vi "Main UI.vi"() -> ()   [LabVIEW 2017]
uses:
  UI typedefs/Controller Commands.ctl
  UI typedefs/Progress States.ctl
  Application Utilities/Console Log/Console Log.lvclass
  Procedure Classes/Potting Procedure/Potting Procedure.lvclass
  Shared Components/Gantry Class/Gantry Class.lvclass
  C:/Program Files/National Instruments/LabVIEW 2017/user.lib/aerotech/2010/Bin/Aerotech.A3200.dll
  Program Files/National Instruments/LabVIEW 2017/user.lib/aerotech/2010/Bin/Aerotech.A3200.dll
  Shared Components/WorkTable Class/Type Definitions/Worktable_Mode.ctl
  Shared Components/Gantry Class/Type Definitions/Virtual Modes.ctl
  UI typedefs/Progress Bar.ctl
panel:
  in  "ESTOP References":T1
  out "Progress":T2 scale=0.0..9.0
  in  "Execute Step":bool
  in  "Resume Button":bool
  in  "Suspend Button":bool
  in  "Add Comment":bool
  in  "Comment":string
  in  "Previous Button":bool
  in  "Manual Control":bool
  in  "Emergency Stop":bool
  out "Console":string
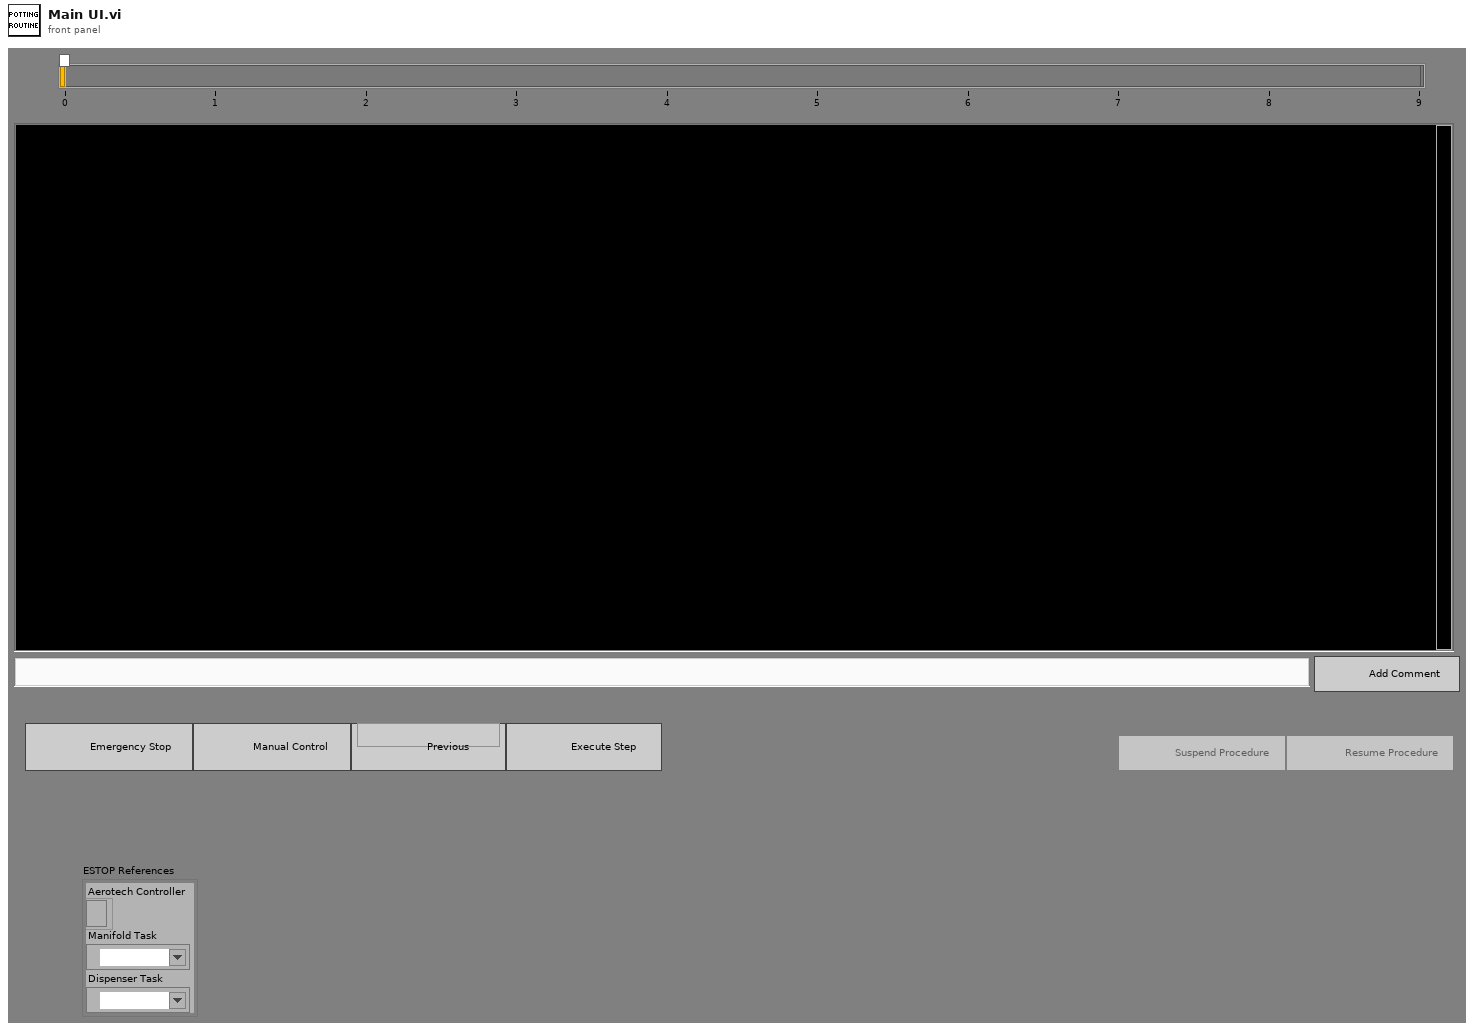
[diagram p1: front panel]
types:
  T1 = cluster{"Aerotech Controller":refnum<k24>, "Manifold Task":refnum<k21>, "Dispenser Task":refnum<k21>}
  T2 = typedef "Progress Bar.ctl" = u16
  T3 = typedef "Progress States.ctl" = enum16{"Configure Tester", "Inspect Fiducials", "Review Fiducials", "Inspect Modules", "Review Modules", "Fill Sylgard", "Align Needle", "Purge", "Pot", "Finish"}
  T4 = typedef "Controller Commands.ctl" = enum16{"Initialize", "Execute Step", "Previous Step", "Add Comment", "Manual Control", "Resume", "Pause", "Emergency Stop"}
  T5 = typedef "Virtual Modes.ctl" = enum16{"Nonvirtual", "Virtual"}
  T6 = typedef "Worktable_Mode.ctl" = enum16{"Encapsulation", "Gluing"}
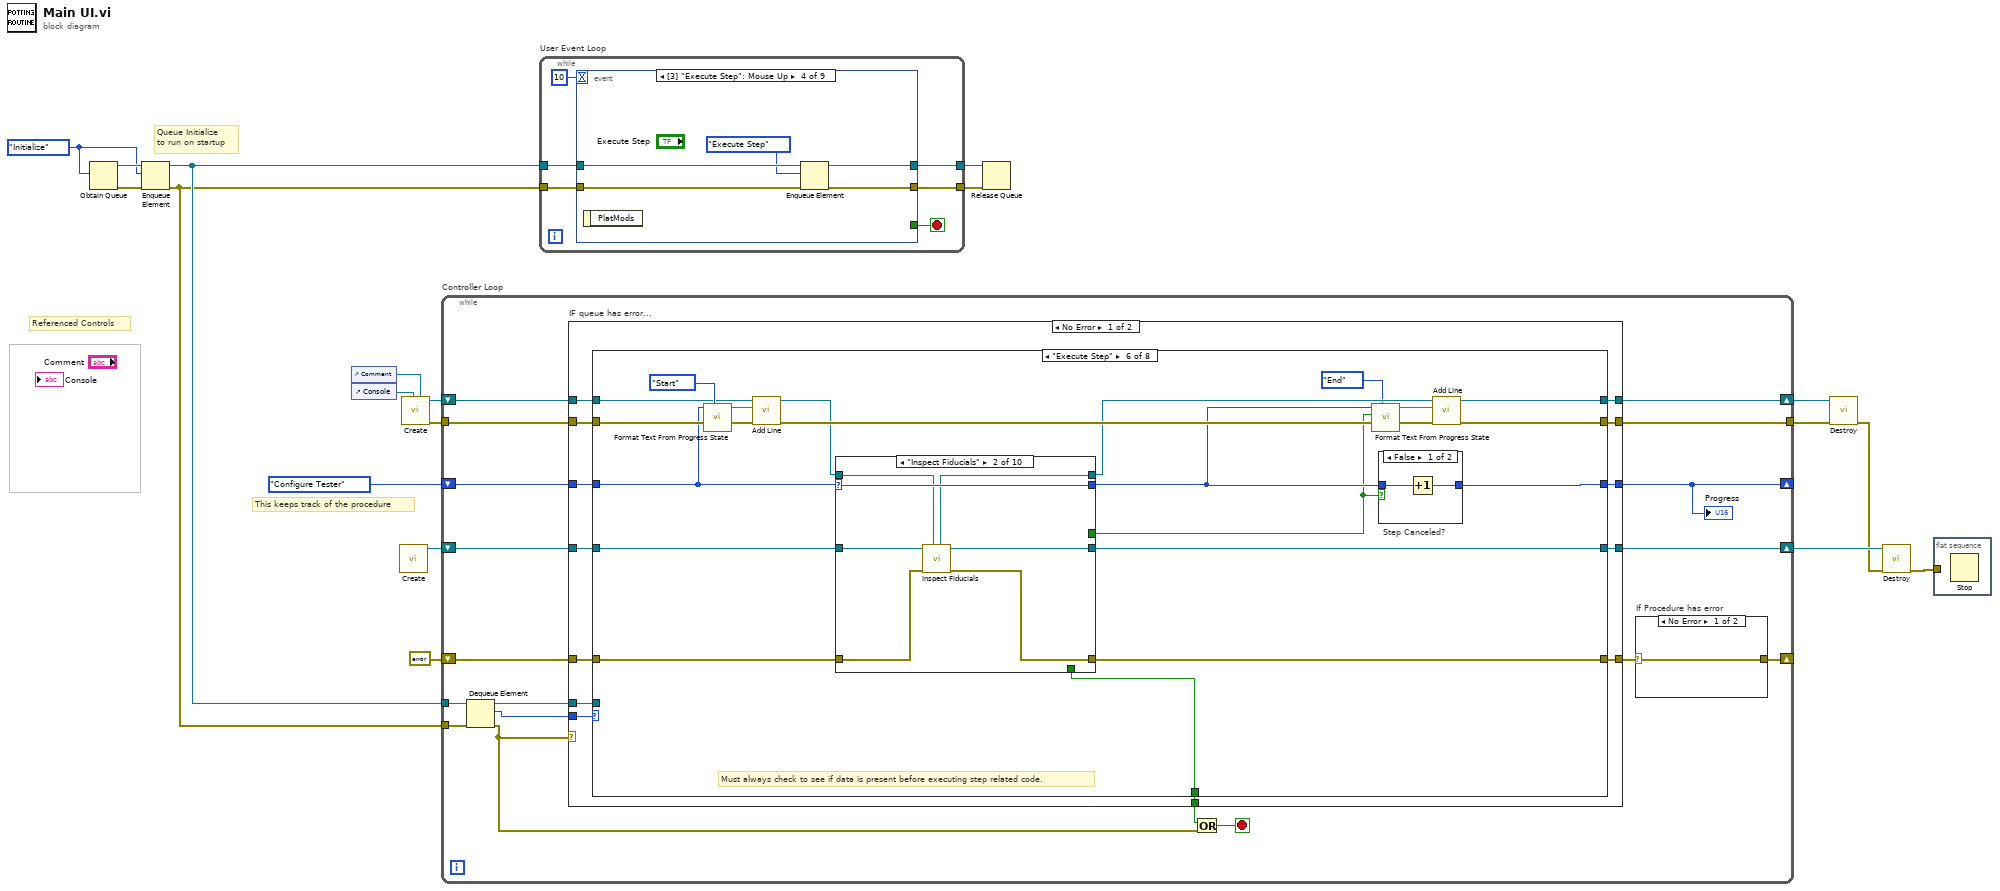
[diagram p0: block diagram]
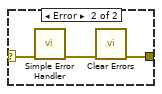
[diagram p2: hidden frame]
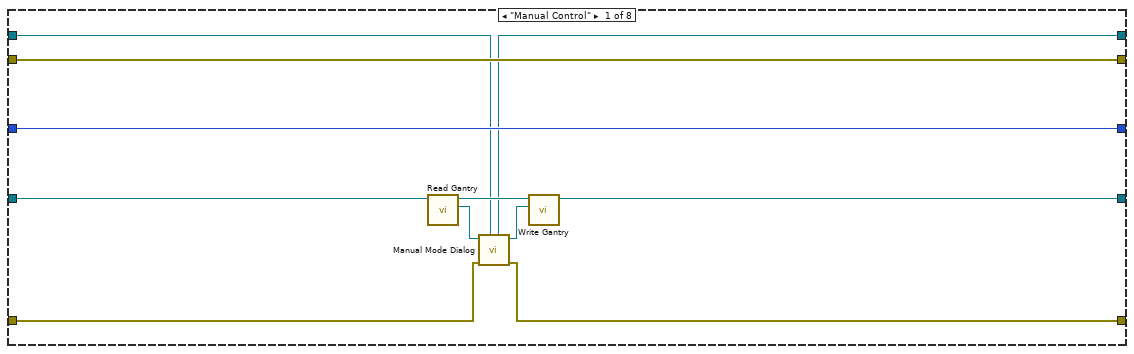
[diagram p3: hidden frame]
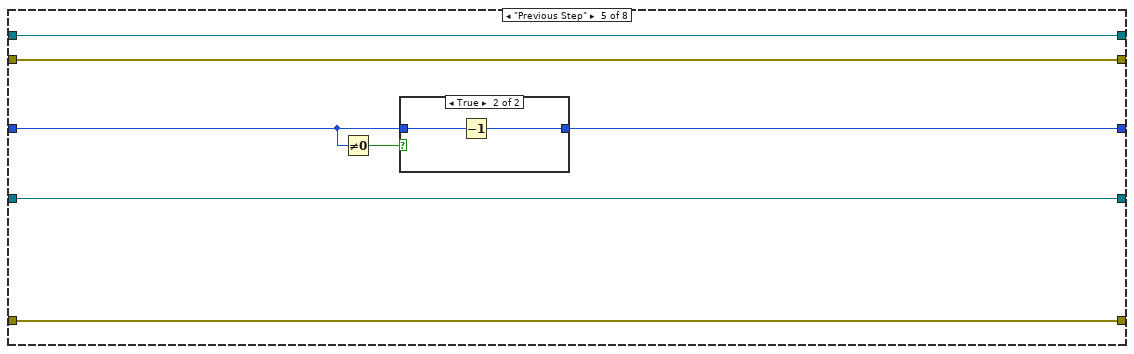
[diagram p7: hidden frame]
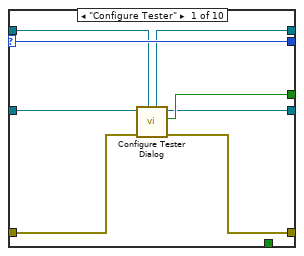
[diagram p10: hidden frame]
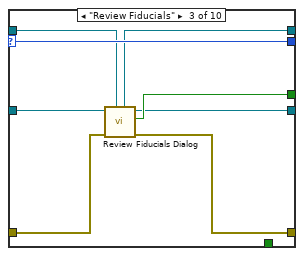
[diagram p11: hidden frame]
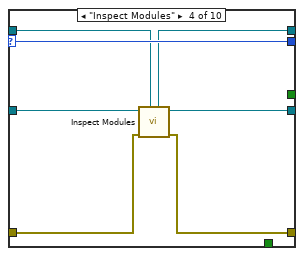
[diagram p12: hidden frame]
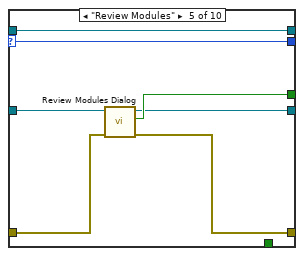
[diagram p13: hidden frame]
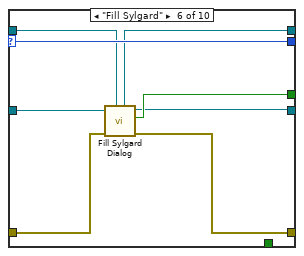
[diagram p14: hidden frame]
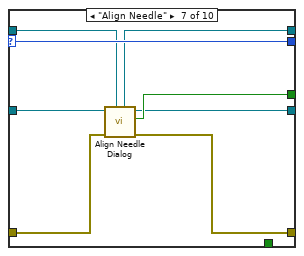
[diagram p15: hidden frame]
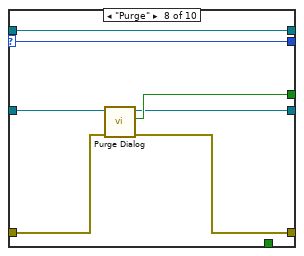
[diagram p16: hidden frame]
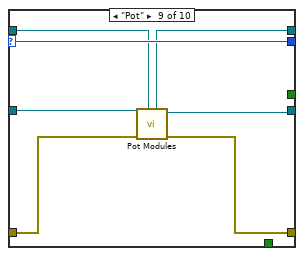
[diagram p17: hidden frame]
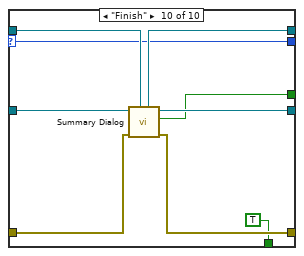
[diagram p18: hidden frame]
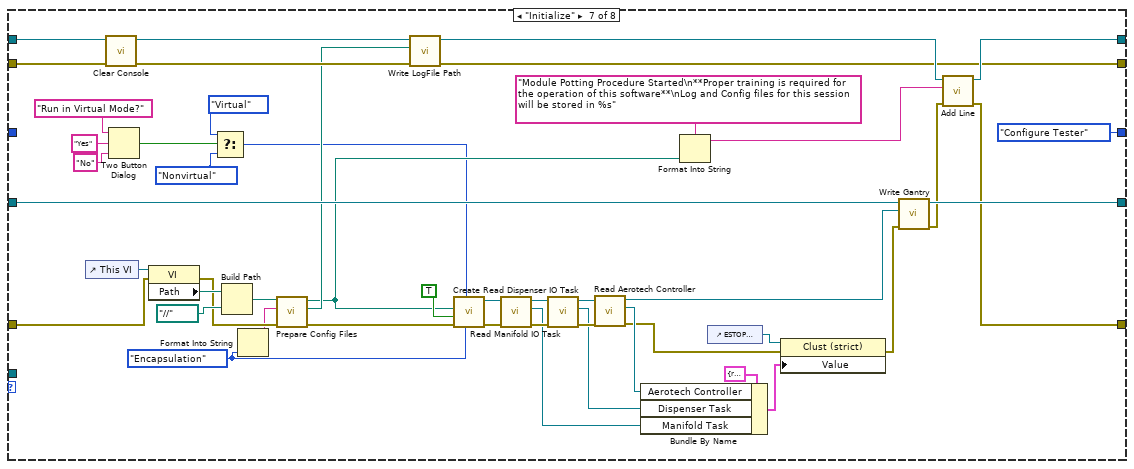
[diagram p19: hidden frame]
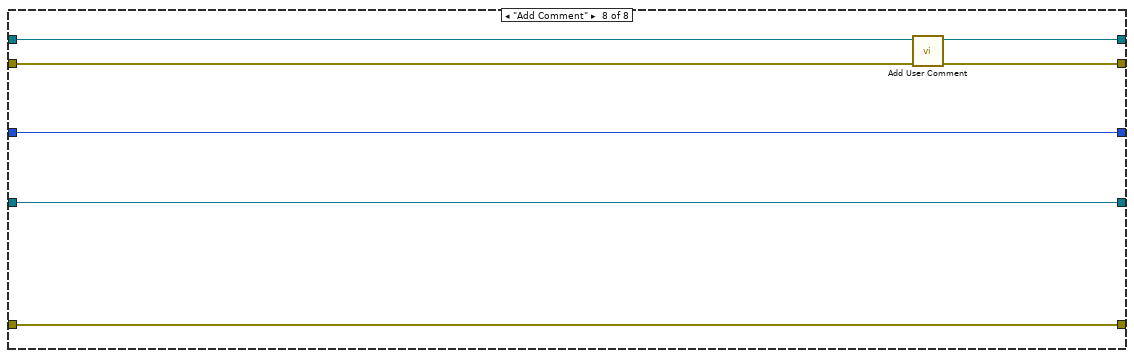
[diagram p20: hidden frame]
diagram:
  w12 = Controller_Commands."Initialize" ("Commands")
  # "Referenced Controls"
  # "This keeps track of the procedure"
  # "Queue Initialize \nto run on startup"
  n1 = Obtain Queue(element data type=w12) -> (queue out=w15:refnum<queue>, error out=w13:errorcluster)  [unwired: 4 in, 1 out]
  n2 = Enqueue Element(queue=w15, element=w12, error in (no error)=w13) -> (queue out=w14:refnum<queue>, error out=w1:errorcluster)  [unwired: 1 in, 1 out]
  n3 = control-ref of="Comment"() -> (w10:refnum<vi>)
  n4 = control-ref of="Console"() -> (w11:refnum<vi>)
  n5 = call "Create.vi"() -> ("Potting Procedure out"=w5:refnum<class "Potting Procedure.lvclass">)  [unwired: 10 in, 1 out]
  n6 = call "Create.vi"("Comment"=w10, "Console"=w11) -> ("error out"=w8:errorcluster, "Console Log out"=w9:refnum<class "Console Log.lvclass">)  [unwired: 8 in]
  n7 = while "Controller Loop" {
    tunnel: w1 -> [w37]
    shift-right: [w20] -> _
    shift-left: Progress_States."Configure Tester" -> [w35]
    tunnel: w14 -> [w34]
    shift-right: [w30] -> _
    shift-left: errorcluster {"status"=FALSE, "code"=0, "source"=""} ("error constant") -> [w32]
    tunnel: w8 -> [w27]
    tunnel: [w26] -> w6
    shift-right: [w28] -> w7
    shift-left: w9 -> [w29]
    shift-right: [w24] -> w4
    shift-left: w5 -> [w25]
    stop <- w22 stop-if-true
    n8 = Dequeue Element(queue=w34, error in (no error)=w37) -> (queue out=w36:refnum<queue>, element=w33:T4, error out=w23:errorcluster)  [unwired: 1 in, 1 out]
    n9 = case "IF queue has error..." shown="No Error" w23 {
      tunnel: w36 -> [w54 _]
      tunnel: w35 -> [w53 w248]
      tunnel: [w52 w248] -> w20
      tunnel: w33 -> [w51 _]
      tunnel: w32 -> [w50 w247]
      tunnel: [w49 w247] -> w31
      tunnel: w29 -> [w48 w246]
      tunnel: [w47 w246] -> w28
      tunnel: w27 -> [w46 w245]
      tunnel: [w45 w245] -> w26
      tunnel: [w43 w244] -> w24
      tunnel: w25 -> [w44 w244]
      tunnel: [w42 _] -> w21
      frame No Error {
        n10 = case shown="\"Execute Step\"" w51 {
          tunnel: w54 -> [_ _ _ _ _ _ _ _]
          tunnel: w53 -> [w65 w70 w75 w80 w82 w92 _ w243]
          tunnel: [w65 w70 w75 w80 w86 w109 Progress_States."Configure Tester" w243] -> w52
          tunnel: w50 -> [w63 w69 w74 w79 w87 w99 w200 w238]
          tunnel: [w62 w69 w74 w79 w87 w98 w210 w238] -> w49
          tunnel: w48 -> [w56 w67 w73 w78 w85 w94 w235 w240]
          tunnel: [w55 w67 w73 w78 w85 w108 w212 w242] -> w47
          tunnel: w46 -> [w64 w68 w72 w77 w84 w107 w234 w239]
          tunnel: [w64 w68 w72 w77 w84 w106 w206 w241] -> w45
          tunnel: w44 -> [w59 w66 w71 w76 w83 w103 w233 w237]
          tunnel: [w57 w66 w71 w76 w83 w102 w232 w237] -> w43
          tunnel: [_ _ _ _ _ w100 _ _] -> w42
          frame "Manual Control" {
            n11 = call-dynamic "Read Gantry.vi"("Potting Procedure in"=w59) -> ("Gantry"=w61:refnum<class "Gantry Class.lvclass">, "Potting Procedure out"=w58:refnum<class "Potting Procedure.lvclass">)  [unwired: 8 in, 1 out]
            n12 = call "Manual Mode Dialog.vi"("Console Log in"=w56, "error in"=w63, "Gantry in"=w61) -> ("error out"=w62:errorcluster, "Gantry out"=w60:refnum<class "Gantry Class.lvclass">, "Console Log out"=w55:refnum<class "Console Log.lvclass">)  [unwired: 6 in]
            n13 = call-dynamic "Write Gantry.vi"("Gantry"=w60, "Potting Procedure in"=w58) -> ("Potting Procedure out"=w57:refnum<class "Potting Procedure.lvclass">)  [unwired: 8 in, 1 out]
          }
          frame "Resume" {
            # "Resume will open some sort of file and restore a procedure."
          }
          frame "Pause" {
            # "Pause will cache the state of a procedure to some sort of file."
          }
          frame "Emergency Stop" {
            # "Any actions resultant of an emergency stop goes here."
          }
          frame "Previous Step" {
            n14 = Not Equal To 0?(x=w82) -> (x != 0?=w81:bool)
            n15 = case shown="True" w81 {
              tunnel: w82 -> [w88 w90]
              tunnel: [w88 w89] -> w86
              frame False {
              }
              frame True {
                n16 = Decrement(x=w90) -> (x-1=w89:T3)
              }
            }
          }
          frame "Execute Step" {
            # "Must always check to see if data is present before executing step related code."
            n17 = call "Format Text From Progress State.vi"("Start/End"=enum16{"Start", "End"}."Start", "Potting Progress States"=w92) -> ("String"=w95:string)  [unwired: 9 in]
            n18 = call "Add Line.vi"("String"=w95, "Console Log in"=w94) -> ("Console Log out"=w93:refnum<class "Console Log.lvclass">)  [unwired: 8 in, 1 out]
            n19 = case shown="\"Inspect Fiducials\"" w92 {
              selector: w92 -> [w118 w127 w135 w142 w149 w157 w165 w172 w179 w181]
              tunnel: [w118 w127 w135 w142 w149 w157 w165 w172 w179 w181] -> w105
              tunnel: w99 -> [w120 w124 w134 w137 w148 w156 w164 w171 w176 w184]
              tunnel: [w119 w123 w133 w136 w147 w155 w163 w170 w175 w183] -> w98
              tunnel: [w117 _ w132 _ w146 w154 w162 w169 _ w182] -> w104
              tunnel: w103 -> [w116 w126 w131 w141 w144 w153 w161 w167 w178 w188]
              tunnel: [w115 w125 w130 w140 w143 w152 w160 w166 w177 w187] -> w102
              tunnel: w93 -> [w114 w122 w129 w139 w145 w151 w159 w168 w174 w186]
              tunnel: [w113 w121 w128 w138 w145 w150 w158 w168 w173 w185] -> w101
              tunnel: [_ _ _ _ _ _ _ _ _ TRUE] -> w100
              frame "Configure Tester" {
                n20 = call "Configure Tester Dialog.vi"("Console Log in"=w114, "error in"=w120, "Potting Procedure In"=w116) -> ("error out"=w119:errorcluster, "Canceled"=w117:bool, "Potting Procedure Out"=w115:refnum<class "Potting Procedure.lvclass">, "Console Log out"=w113:refnum<class "Console Log.lvclass">)  [unwired: 5 in]
              }
              frame "Inspect Fiducials" {
                n21 = call-dynamic "Inspect Fiducials.vi"("Console Log in"=w122, "error in"=w124, "Potting Procedure in"=w126) -> ("error out"=w123:errorcluster, "Potting Procedure out"=w125:refnum<class "Potting Procedure.lvclass">, "Console Log out"=w121:refnum<class "Console Log.lvclass">)  [unwired: 6 in]
              }
              frame "Review Fiducials" {
                n22 = call "Review Fiducials Dialog.vi"("Console Log in"=w129, "error in"=w134, "Potting Procedure in"=w131) -> ("error out"=w133:errorcluster, "Canceled"=w132:bool, "Potting Procedure out"=w130:refnum<class "Potting Procedure.lvclass">, "Console Log out"=w128:refnum<class "Console Log.lvclass">)  [unwired: 5 in]
              }
              frame "Inspect Modules" {
                n23 = call-dynamic "Inspect Modules.vi"("Console Log in"=w139, "error in"=w137, "Potting Procedure in"=w141) -> ("error out"=w136:errorcluster, "Potting Procedure out"=w140:refnum<class "Potting Procedure.lvclass">, "Console Log out"=w138:refnum<class "Console Log.lvclass">)  [unwired: 6 in]
              }
              frame "Review Modules" {
                n24 = call "Review Modules Dialog.vi"("error in"=w148, "Potting Procedure in"=w144) -> ("error out"=w147:errorcluster, "Canceled"=w146:bool, "Potting Procedure out"=w143:refnum<class "Potting Procedure.lvclass">)  [unwired: 7 in]
              }
              frame "Fill Sylgard" {
                n25 = call "Fill Sylgard Dialog.vi"("Console Log in"=w151, "error in"=w156, "Potting Procedure in"=w153) -> ("error out"=w155:errorcluster, "Canceled"=w154:bool, "Potting Procedure out"=w152:refnum<class "Potting Procedure.lvclass">, "Console Log out"=w150:refnum<class "Console Log.lvclass">)  [unwired: 5 in]
              }
              frame "Align Needle" {
                n26 = call "Align Needle Dialog.vi"("Console Log in"=w159, "error in"=w164, "Potting Procedure in"=w161) -> ("error out"=w163:errorcluster, "Canceled"=w162:bool, "Potting Procedure out"=w160:refnum<class "Potting Procedure.lvclass">, "Console Log out"=w158:refnum<class "Console Log.lvclass">)  [unwired: 5 in]
              }
              frame "Purge" {
                n27 = call "Purge Dialog.vi"("error in"=w171, "Potting Procedure in"=w167) -> ("error out"=w170:errorcluster, "Canceled"=w169:bool, "Potting Procedure out"=w166:refnum<class "Potting Procedure.lvclass">)  [unwired: 7 in]
              }
              frame "Pot" {
                n28 = call "Pot Modules.vi"("Console Log in"=w174, "error in"=w176, "Potting Procedure in"=w178) -> ("error out"=w175:errorcluster, "Potting Procedure out"=w177:refnum<class "Potting Procedure.lvclass">, "Console Log out"=w173:refnum<class "Console Log.lvclass">)  [unwired: 6 in]
              }
              frame "Finish" {
                n29 = call "Summary Dialog.vi"("Console Log in"=w186, "error in"=w184, "Potting Procedure in"=w188) -> ("error out"=w183:errorcluster, "Canceled"=w182:bool, "Potting Procedure out"=w187:refnum<class "Potting Procedure.lvclass">, "Console Log out"=w185:refnum<class "Console Log.lvclass">)  [unwired: 5 in]
              }
            }
            n30 = call "Format Text From Progress State.vi"("Start/End"=enum16{"Start", "End"}."End", "Canceled"=w104, "Potting Progress States"=w105) -> ("String"=w96:string)  [unwired: 8 in]
            n31 = case "Step Canceled?" shown="False" w104 {
              tunnel: w105 -> [w111 w112]
              tunnel: [w110 w112] -> w109
              frame False {
                n32 = Increment(x=w111) -> (x+1=w110:T3)
              }
              frame True {
              }
            }
            n33 = call "Add Line.vi"("error in"=w107, "String"=w96, "Console Log in"=w101) -> ("error out"=w106:errorcluster, "Console Log out"=w108:refnum<class "Console Log.lvclass">)  [unwired: 7 in]
          }
          frame "Initialize" {
            w195 = Worktable_Mode."Encapsulation" ("Worktable Mode")
            n34 = control-ref of="This VI"() -> (w205:refnum<vi>)
            n35 = call "Clear Console.vi"("error in (no error)"=w234, "Console Log in"=w235) -> ("error out"=w207:errorcluster, "Console Log out"=w209:refnum<class "Console Log.lvclass">)  [unwired: 8 in]
            n36 = Two Button Dialog(message="Run in Virtual Mode?" ("T button name (\"OK\")"), 1:"No" ("F button name (\"Cancel\")"), 2:"Yes" ("T button name (\"OK\")")) -> (T button?=w192:bool)
            n37 = property class="VI"(reference=w205, error in=w200) -> (error out=w199:errorcluster, "Path"=w204:path)  [unwired: 1 out]
            n38 = Select(t=Virtual_Modes."Virtual" ("Virtual Mode"), s=w192, f=Virtual_Modes."Nonvirtual" ("Virtual Mode")) -> (s? t:f=w189:T5)
            n39 = Build Path(base path=w204, name or relative path=path "../../..") -> (appended path=w201:path)
            n40 = Format Into String(w195) -> (resulting string=w196:string)  [unwired: 3 in, 1 out]
            n41 = call "Prepare Config Files.vi"("error in"=w199, "Config Prefix"=w196, "Project Root"=w201) -> ("error out"=w202:errorcluster, "Log Directory"=w194:path, "Config Directory"=w193:path)  [unwired: 6 in]
            n42 = call-dynamic "Write LogFile Path.vi"("error in"=w207, "Log Filename"=w194, "Console Log in"=w209) -> ("error out"=w206:errorcluster, "Console Log out"=w208:refnum<class "Console Log.lvclass">)  [unwired: 7 in]
            n43 = call "Create.vi"(6:w195, "Virtual Mode"=w189, "error in"=w202, "HOME?"=TRUE, "Config Folder"=w193) -> ("error out"=w220:errorcluster, "Gantry out"=w224:refnum<class "Gantry Class.lvclass">)  [unwired: 5 in]
            n44 = call-dynamic "Read Manifold IO Task.vi"("error in (no error)"=w220, "Gantry Class in"=w224) -> ("error out"=w219:errorcluster, "Manifold IO Task"=w217:refnum<k21>, "Gantry Class out"=w223:refnum<class "Gantry Class.lvclass">)  [unwired: 7 in]
            n45 = call-dynamic "Read Dispenser IO Task.vi"("error in (no error)"=w219, "Gantry Class in"=w223) -> ("error out"=w218:errorcluster, "Dispenser IO Task"=w216:refnum<k21>, "Gantry Class out"=w222:refnum<class "Gantry Class.lvclass">)  [unwired: 7 in]
            n46 = call-dynamic "Read Aerotech Controller.vi"("error in (no error)"=w218, "Gantry Class in"=w222) -> ("error out"=w214:errorcluster, "Aerotech Controller"=w215:refnum<k24>, "Gantry Class out"=w221:refnum<class "Gantry Class.lvclass">)  [unwired: 7 in]
            n47 = Bundle By Name(cluster=T1 {"Aerotech Controller"=refnum, "Manifold Task"="", "Dispenser Task"=""} ("Value"), "Aerotech Controller"=w215, "Dispenser Task"=w216, "Manifold Task"=w217) -> (w225:T1)
            n48 = Format Into String(format string="Module Potting Procedure Started\n**Proper training is required for the operation of this software**\nLog and Config files for this session will be stored in %s" ("String"), w193) -> (resulting string=w197:string)  [unwired: 2 in, 1 out]
            n49 = control-ref of="ESTOP References"() -> (w227:refnum<vi>)
            n50 = property class="Clust (strict)"(reference=w227, error in=w214, "Value"=w225) -> (error out=w213:errorcluster)  [unwired: 1 out]
            n51 = call-dynamic "Write Gantry.vi"("error in (no error)"=w213, "Gantry"=w221, "Potting Procedure in"=w233) -> ("error out"=w211:errorcluster, "Potting Procedure out"=w232:refnum<class "Potting Procedure.lvclass">)  [unwired: 7 in]
            n52 = call "Add Line.vi"("error in"=w211, "String"=w197, "Console Log in"=w208) -> ("error out"=w210:errorcluster, "Console Log out"=w212:refnum<class "Console Log.lvclass">)  [unwired: 7 in]
          }
          frame "Add Comment" {
            n53 = call "Add User Comment.vi"("error in"=w239, "Console Log in"=w240) -> ("error out"=w241:errorcluster, "Console Log out"=w242:refnum<class "Console Log.lvclass">)  [unwired: 8 in]
          }
        }
      }
      frame Error {
      }
    }
    "Progress" <- w20
    n54 = Or(x=w21, y=w23) -> (x .or. y?=w22:bool)
    n55 = case "If Procedure has error" shown="No Error" w31 {
      selector: w31 -> [w38 w41]
      tunnel: [w38 w40] -> w30
      frame No Error {
      }
      frame Error {
        n56 = call <vilib>:"Simple Error Handler.vi"("error in (no error)"=w41) -> ("error out"=w39:errorcluster)  [unwired: 4 in, 4 out]
        n57 = call <vilib>:"Clear Errors.vi"("error in (no error)"=w39) -> ("error out"=w40:errorcluster)  [unwired: 5 in, 1 out]
      }
    }
  }
  n58 = while "User Event Loop" {
    tunnel: w14 -> [w249]
    tunnel: [w252] -> w19
    tunnel: w1 -> [w251]
    tunnel: [w250] -> w18
    stop <- w253 stop-if-true
    n59 = event shown="[3] \"Execute Step\": Mouse Up" {
      selector: _ -> [_ _ _ _ _ _ _ _ _]
      dyn-events: _ -> [_ _ _ _ _ _ _ _ _]
      timeout: 10 -> [_ _ _ _ _ _ _ _ _]
      tunnel: [_ _ _ _ _ _ _ w281 _] -> w253
      tunnel: w249 -> [w256 w259 w263 w269 w271 w276 w278 w280 w287]
      tunnel: [w256 w259 w262 w266 w273 w276 w278 w280 w288] -> w252
      tunnel: w251 -> [w255 w258 w261 w268 w270 w275 w277 w279 w290]
      tunnel: [w255 w258 w260 w267 w272 w275 w277 w279 w289] -> w250
      event Timeout {
        n60 = event-data() -> ()  [unwired: 1 in, 1 out]
      }
      event "Emergency Stop": Mouse Up {
        n61 = event-data() -> ()  [unwired: 1 in, 1 out]
        n62 = call "Emergency Stop.vi"("ESTOP References"="ESTOP References") -> ()
      }
      event "Manual Control": Mouse Up {
        n63 = event-data() -> ()  [unwired: 1 in, 1 out]
        n64 = Enqueue Element(queue=w263, element=Controller_Commands."Manual Control", error in (no error)=w261) -> (queue out=w262:refnum<queue>, error out=w260:errorcluster)  [unwired: 1 in, 1 out]
      }
      event "Execute Step": Mouse Up {
        n65 = event-data() -> ()  [unwired: 1 in, 1 out]
        n66 = Enqueue Element(queue=w269, element=Controller_Commands."Execute Step", error in (no error)=w268) -> (queue out=w266:refnum<queue>, error out=w267:errorcluster)  [unwired: 1 in, 1 out]
      }
      event "Previous Button": Mouse Up {
        n67 = event-data() -> ()  [unwired: 1 in, 1 out]
        n68 = Enqueue Element(queue=w271, element=Controller_Commands."Previous Step", error in (no error)=w270) -> (queue out=w273:refnum<queue>, error out=w272:errorcluster)  [unwired: 1 in, 1 out]
      }
      event "Suspend Button": Mouse Up {
        n69 = event-data() -> ()  [unwired: 1 in, 1 out]
      }
      event "Resume Button": Mouse Up {
        n70 = event-data() -> ()  [unwired: 1 in, 1 out]
      }
      event Panel Close? {
        n71 = event-data() -> ()  [unwired: 1 in, 1 out]
        n72 = Two Button Dialog(message="Are you sure you want to quit?", 1:"Return" ("F button name (\"Cancel\")"), 2:"Quit" ("T button name (\"OK\")")) -> (T button?=w281:bool)
        n73 = event-data("Discard?"=TRUE) -> ()  [unwired: 1 in, 1 out]
      }
      event "Add Comment": Mouse Up {
        n74 = event-data() -> ()  [unwired: 1 in, 1 out]
        n75 = Enqueue Element(queue=w287, element=Controller_Commands."Add Comment", error in (no error)=w290) -> (queue out=w288:refnum<queue>, error out=w289:errorcluster)  [unwired: 1 in, 1 out]
      }
    }
  }
  n76 = Release Queue(queue=w19, error in (no error)=w18) -> ()  [unwired: 1 in, 3 out]
  n77 = call "Destroy.vi"("error in"=w6, "Console Log in"=w7) -> ("error out"=w2:errorcluster)  [unwired: 9 in]
  n78 = call "Destroy.vi"("error in"=w2, "Potting Procedure in"=w4) -> ("error out"=w3:errorcluster)  [unwired: 9 in]
  n79 = flat-sequence {
    tunnel: w3 -> [_]
    frame #0 {
      n80 = Stop() -> ()  [unwired: 1 in]
    }
  }
